vi "testInternationalCharactersInComment.vi"(8 "error in (no error)":errorcluster, 11 "TestCase in":refnum<class "EasyXMLTest.lvclass">) -> (0 "error out":errorcluster, 3 "TestCase out":refnum<class "EasyXMLTest.lvclass">)   [LabVIEW 2013, in "EasyXMLTest.lvclass"]
doc: "Verify that error in is not overwritten"
uses:
  EasyXMLTest.lvclass
panel:
  out "Produced Data":variant
  out "Input Data":variant
  out "XML String":string
  out "Expected Data":string
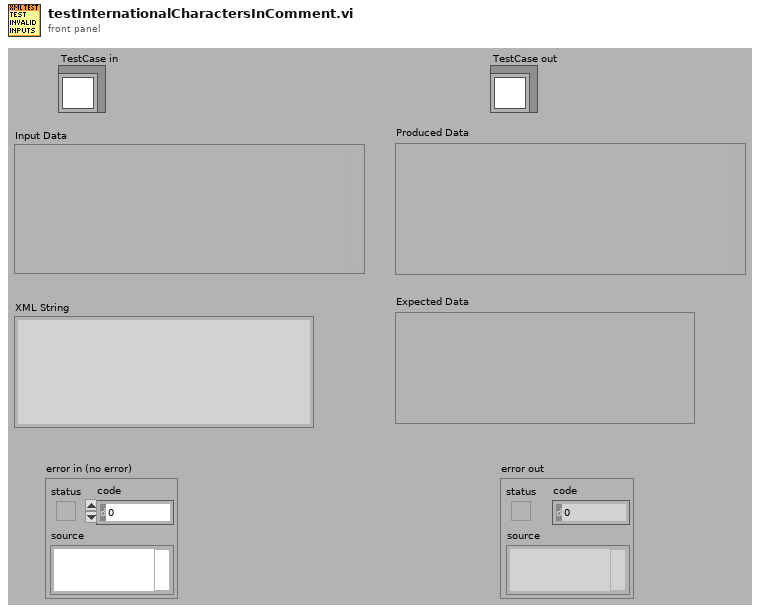
[diagram p1: front panel]
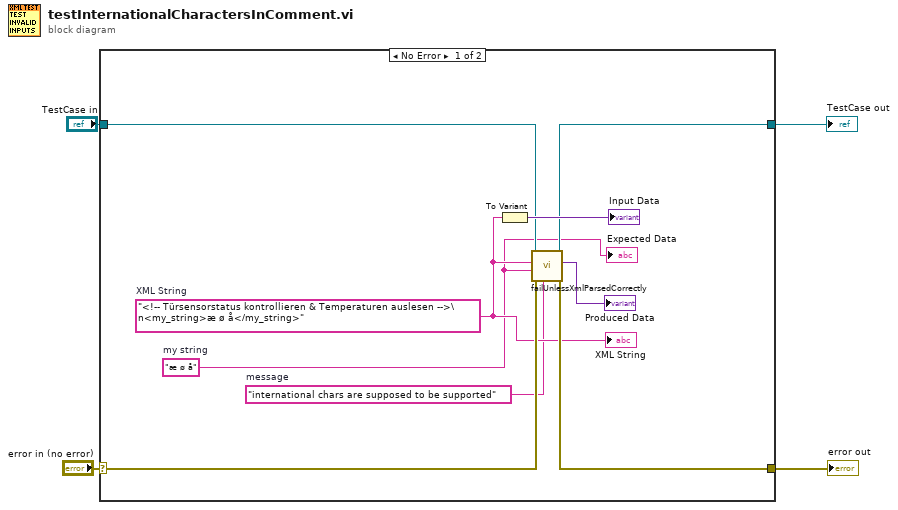
[diagram p0: block diagram]
diagram:
  n1 = case shown="No Error" "error in (no error)" {
    selector: "error in (no error)" -> [w10 w15]
    tunnel: [w9 w15] -> w2
    tunnel: [w11 w14] -> w1
    tunnel: "TestCase in" -> [w12 w14]
    frame No Error {
      w6 = "æ ø å"  # my string
      w7 = "<!-- Türsensorstatus kontrollieren & Temperaturen auslesen -->\n<my_string>æ ø å</my_string>"  # XML String
      w5 = "international chars are supposed to be supported"  # message
      n2 = To Variant(anything=w7) -> (Variant=→"Input Data":variant)
      n3 = call "failUnlessXmlParsedCorrectly.vi"("message (\"\")"=w5, "error in"=w10, "Expected Data"=w6, "XML String"=w7, "reference in"=w12) -> ("error out"=w9:errorcluster, "Produced Data"=→"Produced Data":variant, "reference in"=w11:refnum<class "EasyXMLTest.lvclass">)  [unwired: 4 in]
      "XML String" <- w7
      "Expected Data" <- w6
    }
    frame Error {
    }
  }
  "error out" <- w2
  "TestCase out" <- w1
